vi "Get Frequency.vi"(8 "error in (no error)":errorcluster, 11 "VISA resource name":refnum<visa-resource-name>) -> (0 "error out":errorcluster, 2 "Frequency [Hz]":dbl, 3 "VISA resource name out":refnum<visa-resource-name>)   [LabVIEW 2012, in "Datron D4xxx.lvlib"]
doc: "This VI returns instrument frequency in AC modes."
uses:
  Datron D4xxx.lvlib
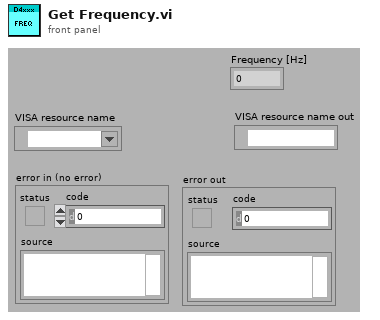
[diagram p1: front panel]
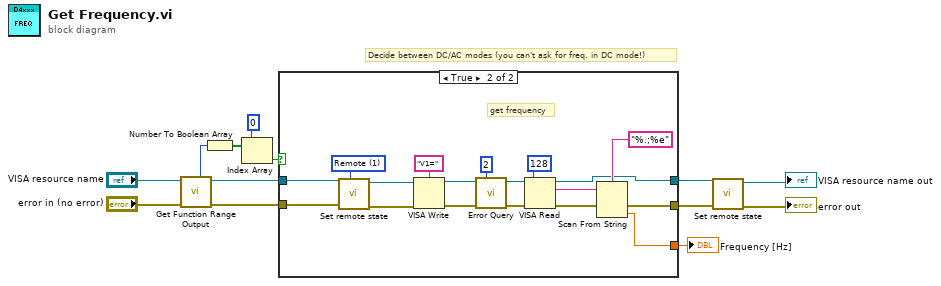
[diagram p0: block diagram]
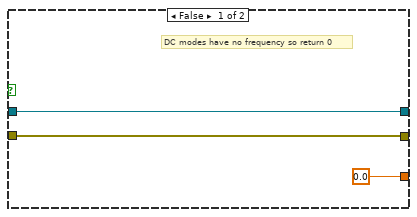
[diagram p2: hidden frame]
diagram:
  # "Decide between DC/AC modes (you can't ask for freq. in DC mode!)"
  n1 = call "Get Function Range Output.vi"("error in (no error)"="error in (no error)", "VISA resource name"="VISA resource name") -> ("error out"=w11:errorcluster, "VISA resource name out"=w5:refnum<visa-resource-name>, "Function {F0-F5}"=w9:i32)  [unwired: 2 in, 5 out]
  n2 = Number To Boolean Array(number=w9) -> (Boolean array=w8:bool[])
  n3 = Index Array(array=w8, index=0) -> (element=w6:bool)
  n4 = case shown="True" w6 {
    tunnel: [w15 w29] -> w4
    tunnel: [w16 w28] -> w1
    tunnel: [0.0 w27] -> w13
    tunnel: w11 -> [w15 w21]
    tunnel: w5 -> [w16 w19]
    frame False {
      # "DC modes have no frequency so return 0"
    }
    frame True {
      w17 = u16 1 items=["Local", "Remote", "Default"] ("Remote state")
      # "get frequency"
      n5 = call "Set remote state.vi"("error in"=w21, "Remote state"=w17, "VISA resource name"=w19) -> ("error out"=w20:errorcluster, "VISA resource name out"=w18:refnum<visa-resource-name>)  [unwired: 7 in]
      n6 = VISA Write(VISA resource name=w18, write buffer="V1=", error in (no error)=w20) -> (VISA resource name out=w24:refnum<visa-resource-name>, error out=w23:errorcluster)  [unwired: 1 out]
      n7 = call "Error Query.vi"("error in (no error)"=w23, "Check cycles (11)"=2, "VISA resource name"=w24) -> ("error out"=w26:errorcluster, "VISA resource name out"=w25:refnum<visa-resource-name>)  [unwired: 5 in, 2 out]
      n8 = VISA Read(VISA resource name=w25, byte count=u32 128, error in (no error)=w26) -> (VISA resource name out=w28:refnum<visa-resource-name>, read buffer=w30:string, error out=w32:errorcluster)  [unwired: 1 out]
      n9 = Scan From String(format string="%.;%e", input string=w30, error in=w32) -> (error out=w29:errorcluster, output 1=w27:dbl)  [unwired: 2 in, 2 out]
    }
  }
  "Frequency [Hz]" <- w13
  n10 = call "Set remote state.vi"("error in"=w4, "VISA resource name"=w1) -> ("error out"=→"error out":errorcluster, "VISA resource name out"=→"VISA resource name out":refnum<visa-resource-name>)  [unwired: 8 in]
